vi "queue sm 3.vi"() -> ()   [LabVIEW 2021]
uses:
  file I O/ASSIGN 8/que sm states.ctl
panel:
  out "data":i32[][](array[numeric])
  out "State output":string
  out "state":T1
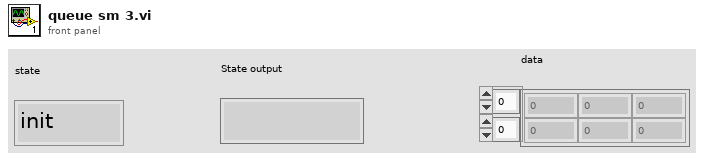
[diagram p1: front panel]
types:
  T1 = typedef "que sm states.ctl" = enum16{"init", "events", "state 1", "state 2", "stop"}
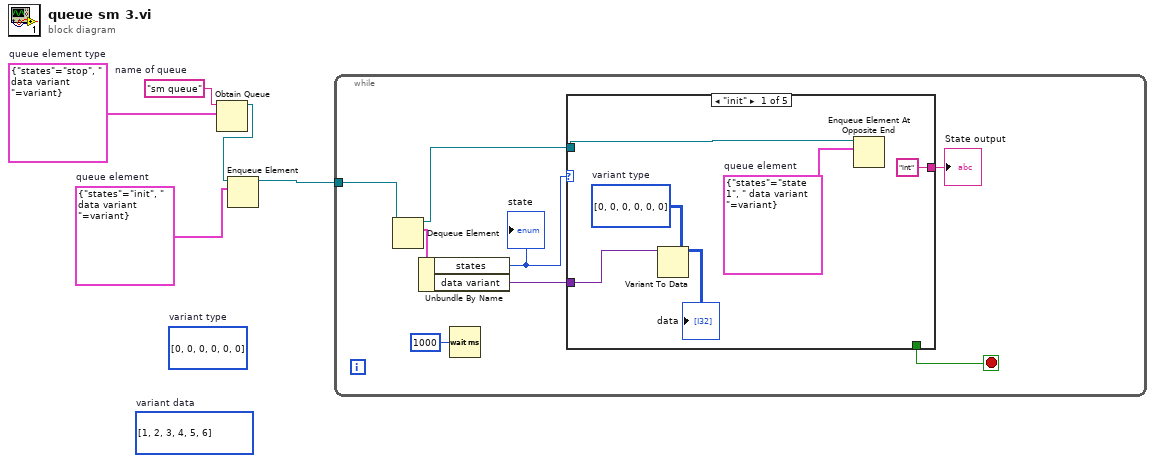
[diagram p0: block diagram]
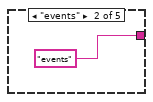
[diagram p2: hidden frame]
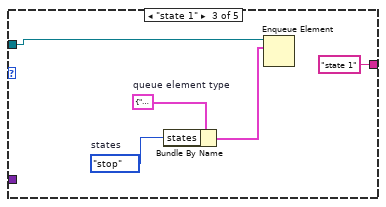
[diagram p3: hidden frame]
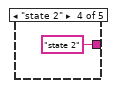
[diagram p4: hidden frame]
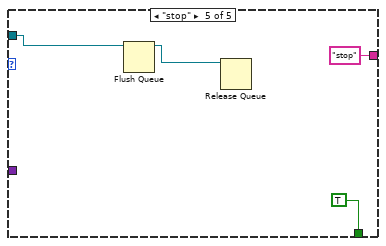
[diagram p5: hidden frame]
diagram:
  w1 = cluster{"states":T1, " data variant ":variant} {"states"=enum."init", " data variant "=variant(i32[][] [[0, 0, 0], [0, 0, 0]])}  # queue element
  (unwired) i32[][] [[0, 0, 0], [0, 0, 0]]  # variant type
  (unwired) i32[][] [[1, 2, 3], [4, 5, 6]]  # variant data
  w4 = "sm queue"  # name of queue
  w5 = cluster{"states":T1, " data variant ":variant} {"states"=enum."stop", " data variant "=variant(i32[][] [[0, 0, 0], [0, 0, 0]])}  # queue element type
  n1 = Obtain Queue(name (unnamed)=w4, element data type=w5) -> (queue out=w3:refnum<queue>)  [unwired: 3 in, 2 out]
  n2 = Enqueue Element(queue=w3, element=w1) -> (queue out=w2:refnum<queue>)  [unwired: 2 in, 2 out]
  n3 = while {
    tunnel: w2 -> [w10]
    stop <- w7 stop-if-true
    n4 = Dequeue Element(queue=w10) -> (queue out=w9:refnum<queue>, element=w13:cluster{"states":T1, " data variant ":variant})  [unwired: 2 in, 2 out]
    n5 = Unbundle By Name(w13) -> ("states"=w8:T1, "data variant"=w6:variant)
    "state" <- w8
    n6 = Wait (ms)(milliseconds to wait=u32 1000) -> ()  [unwired: 1 out]
    n7 = case shown="\"init\"" w8 {
      tunnel: w9 -> [w19 _ w24 _ w28]
      tunnel: ["int" "events" "state 1" "state 2" "stop"] -> w11
      tunnel: [_ _ _ _ TRUE] -> w7
      tunnel: w6 -> [w14 _ _ _ _]
      frame "init" {
        w15 = cluster{"states":T1, " data variant ":variant} {"states"=enum."state 1", " data variant "=variant(i32[][] [[0, 0, 0], [0, 0, 0]])}  # queue element
        w17 = i32[][] [[0, 0, 0], [0, 0, 0]]  # variant type
        n8 = Variant To Data(type=w17, Variant=w14) -> (data=→"data":i32[][])  [unwired: 1 in, 1 out]
        n9 = Enqueue Element At Opposite End(queue=w19, element=w15) -> ()  [unwired: 2 in, 3 out]
      }
      frame "events" {
      }
      frame "state 1" {
        w21 = cluster{"states":T1, " data variant ":variant} {"states"=enum."stop", " data variant "=variant(i32[][] [[0, 0, 0], [0, 0, 0]])}  # queue element type
        w23 = que_sm_states."stop"  # states
        n10 = Bundle By Name(cluster=w21, "states"=w23) -> (w22:cluster{"states":T1, " data variant ":variant})
        n11 = Enqueue Element(queue=w24, element=w22) -> ()  [unwired: 2 in, 3 out]
      }
      frame "state 2" {
      }
      frame "stop" {
        n12 = Flush Queue(queue=w28) -> (queue out=w27:refnum<queue>)  [unwired: 1 in, 2 out]
        n13 = Release Queue(queue=w27) -> ()  [unwired: 2 in, 3 out]
      }
    }
    "State output" <- w11
  }
